vi "Close Session.vi"(0 "device session in":refnum<class "Device Session.lvclass">, 11 "error in":errorcluster) -> (15 "error out":errorcluster)   [LabVIEW 2021, in "Device Session.lvclass"]
doc: "Releases allocated memory and closes the session opened with the <B>Open Session</B> VI of this library. This VI closes the session even if <B>error in</B> contains an error.\n\n<B>Input Parameters</B>\n\n<B>device session in</B> is a reference to the Device Session object, which contains a session to each instrument design library used in this sample project. This parameter is obtained from the 'Open Session' VI.\n\n<B>error in</B> describes error conditions that occur before this node runs. This input provides standard 'error in' functionality.\n\n<B>Output Parameters</B>\n\n<B>error out</B> contains error information. This output provides standard 'error out' functionality."
uses:
  Device Session.lvclass
  Device Session.lvclass/Device Session.ctl
  <instrlib>/HSAI-RIO/Config/Group A/v1/Host/Main/niHSAI Group A Config v1 Host.lvclass
  <instrlib>/_niInstr/FIFO Register Bus/v1/Host/niInstr FIFO Register Bus v1 Host.lvclass
  <instrlib>/HSAI-RIO/Cal Data/Interface/v1/Host/Cal Data/niHSAI Cal Data v1 Host.lvclass
  <instrlib>/_niInstr/Instruction Framework/v1/Host/Subsystem Map/niInstr Subsystem Map v1 Host.lvclass
  <instrlib>/_niInstr/Multirecord Acquisition/Interface/v1/Host/niInstr Multirecord Acquisition v1 Host.lvclass
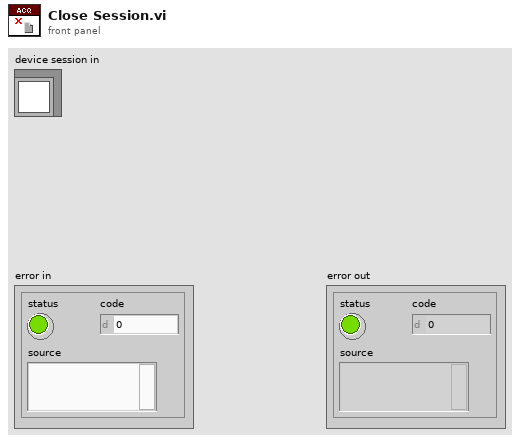
[diagram p1: front panel]
types:
  T1 = typedef "Device Session.lvclass/Device Session Object.ctl" = cluster{"fpga reference":T2, "reg bus":refnum<class "niInstr FIFO Register Bus v1 Host.lvclass">, "subsystem map":refnum<class "niInstr Subsystem Map v1 Host.lvclass">, "cal data":refnum<class "niHSAI Cal Data v1 Host.lvclass">, "config":refnum<class "niHSAI Group A Config v1 Host.lvclass">, "acquisition refs":refnum<class "niInstr Multirecord Acquisition v1 Host.lvclass">[], "acquisition 1":refnum<class "niInstr Multirecord Acquisition v1 Host.lvclass">, "number of selected acq channels":u8, "selected acq channels":bool[], "number of channels":u32, "configured channels":bool[], "acq configuration":cluster{"number of samples":u64, "number of records":u64, "pretrigger samples":u64}, "actual channel configuration":T3[], "sample clock rate (Hz)":dbl, "scaling coefficients":T7[]}
  T2 = typedef "Device Session.lvclass/FPGA Refnum.ctl" = refnum<k20>
  T3 = typedef "niHSAI Types v1 Host.lvlib/Channel Configuration.ctl" = cluster{"channel":u32, "coupling":T4, "impedance":T5, "bandwidth":T6, "vertical range":dbl, "vertical offset":dbl}
  T4 = typedef "niHSAI Types v1 Host.lvlib/Coupling.ctl" = enum8{"Default", "DC", "AC"}
  T5 = typedef "niHSAI Types v1 Host.lvlib/Impedance.ctl" = enum8{"Default", "1 mega ohm", "50 ohm"}
  T6 = typedef "niHSAI Types v1 Host.lvlib/Bandwidth.ctl" = enum8{"Default", "Full Bandwidth", "Anti-alias Filter", "150 MHz"}
  T7 = typedef "niInstr Multirecord Acquisition v1 Host.lvclass/Scaling Coefficient.ctl" = cluster{"gain":dbl, "offset":dbl}
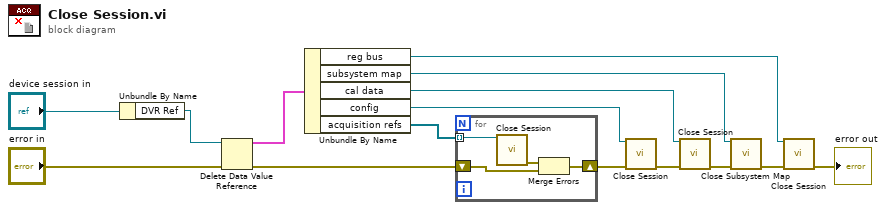
[diagram p0: block diagram]
diagram:
  n1 = Unbundle By Name("device session in") -> ("DVR Ref"=w13:refnum<data-value>)
  n2 = Delete Data Value Reference(data value reference=w13, error in="error in") -> (data value=w12:T1, error out=w11:errorcluster)
  n3 = Unbundle By Name(w12) -> ("reg bus"=w5:refnum<class "niInstr FIFO Register Bus v1 Host.lvclass">, "subsystem map"=w4:refnum<class "niInstr Subsystem Map v1 Host.lvclass">, "cal data"=w3:refnum<class "niHSAI Cal Data v1 Host.lvclass">, "config"=w2:refnum<class "niHSAI Group A Config v1 Host.lvclass">, "acquisition refs"=w1:refnum<class "niInstr Multirecord Acquisition v1 Host.lvclass">[])
  n4 = for {
    tunnel: w1 -> [w18] mode=indexing
    shift-right: [w17] -> w8
    shift-left: w11 -> [w16]
    n5 = call-dynamic "Close Session.vi"("session in"=w18) -> ("error out"=w19:errorcluster)  [unwired: 14 in]
    n6 = Merge Errors(w19, w16) -> (w17:errorcluster)
  }
  n7 = call-dynamic "Close Session.vi"("session in"=w2, "error in"=w8) -> ("error out"=w10:errorcluster)  [unwired: 13 in]
  n8 = call-dynamic "Close Session.vi"("calibration data in"=w3, "error in"=w10) -> ("error out"=w7:errorcluster)  [unwired: 13 in]
  n9 = call-dynamic "Close Subsystem Map.vi"("subsystem map"=w4, "error in"=w7) -> ("error out"=w6:errorcluster)  [unwired: 13 in]
  n10 = call-dynamic "Close Session.vi"("session in"=w5, "error in"=w6) -> ("error out"=→"error out":errorcluster)  [unwired: 13 in]
